vi "Write Log Message.vi"(8 "error in (no error)":errorcluster, 10 "Write Log Message Arguments":T1, 11 "CSV Test Log in":refnum<class "CSV Test Log.lvclass">) -> (0 "error out":errorcluster, 3 "CSV Test Log out":refnum<class "CSV Test Log.lvclass">)   [LabVIEW 2015, in "CSV Test Log.lvclass"]
uses:
  CSV Test Log.lvclass
  Typedefs/Write Log Message Arguments.ctl
  CSV Test Log.lvclass/CSV Test Log.ctl
  Typedefs/FAMT Typedefs.lvlib
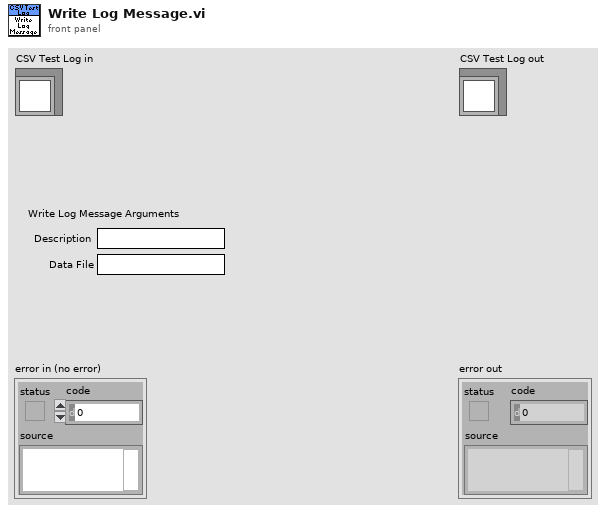
[diagram p1: front panel]
types:
  T1 = typedef "FAMT Typedefs.lvlib/Write Log Message Arguments.ctl" = cluster{"Description":string, "Data File":string}
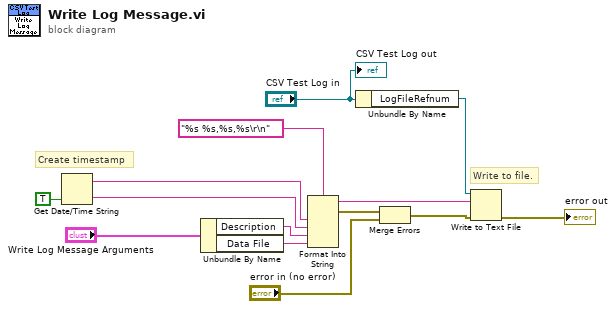
[diagram p0: block diagram]
diagram:
  # "Write to file."
  # "Create timestamp"
  n1 = Get Date/Time String(want seconds? (F)=TRUE) -> (date string=w7:string, time string=w6:string)  [unwired: 2 in]
  n2 = Unbundle By Name("Write Log Message Arguments") -> ("Description"=w5:string, "Data File"=w4:string)
  n3 = Format Into String(format string="%s %s,%s,%s\r\n", w7, w6, w5, w4) -> (resulting string=w3:string, error out=w2:errorcluster)  [unwired: 2 in]
  n4 = Unbundle By Name("CSV Test Log in") -> ("LogFileRefnum"=w12:refnum<file>)
  n5 = Merge Errors(w2, "error in (no error)") -> (w13:errorcluster)
  n6 = Write to Text File(file (use dialog)=w12, text=w3, error in=w13) -> (error out=→"error out":errorcluster)  [unwired: 1 in, 2 out]
  "CSV Test Log out" <- "CSV Test Log in"
